vi "1C Camera Interpreter.vi"() -> (0 "error out":errorcluster, 1 "Overhead Image":T1(plugin-control), 2 "Heading":T2 format="%05.1f", 3 "Boat Location":T3, 4 "Time Elapsed (s)\nSince Last Image":dbl)   [LabVIEW 2011]
doc: "Using data from a cameram, attempts to track two fiducial patterns on the boat, one on the bow and one on the stern. Uses these positions to estimate boat position in the pool.\n\noptimizations for speed: \n-uses an oval-shaped mask to search for the tracking patterns only inside the pool\n-runs the two pattern searches separately so that they can be parallelized\n-upgraded to larger patterns\n\nBy: Cory Dolphin, Jason Curtis, Gray Thomas"
uses:
  <vilib>/userdefined/High Color/IMAQdx.ctl
  2-RIO/2 Typedefs/UTM Location.ctl
  2-RIO/2 Typedefs/heading.ctl
  2-RIO/2 Typedefs/indicator LED.ctl
  2-RIO/2 Globals/2 Global.vi
  <vilib>/vision/driver/NI_Vision_Acquisition_Software.lvlib
panel:
  out "Masked image":T1(plugin-control)
  in  "Minimum Stern Match Score":sgl=650.0
  in  "Minimum Bow Match Score":sgl=850.0
  in  "Reset Camera":bool
  in  "Camera Selector":T4="cam7"
  # "(ignore UTM Zone \nand Hemisphere for \nRC boat)"
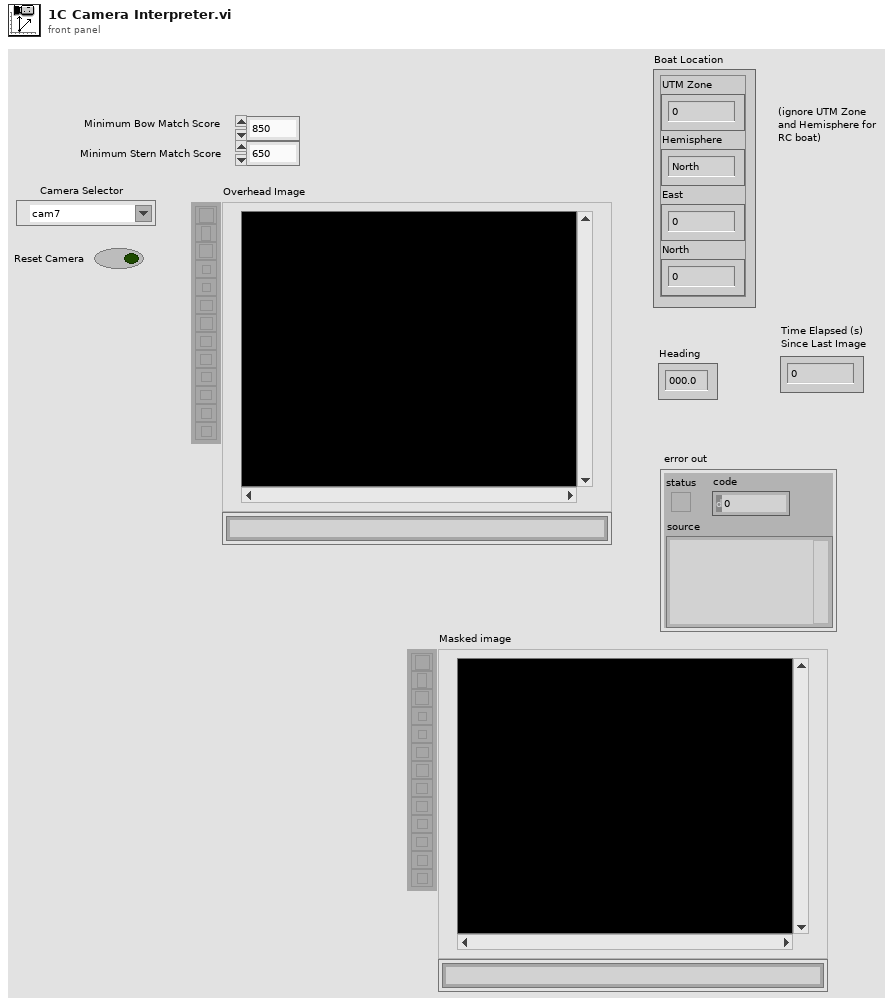
[diagram p1: front panel]
types:
  T1 = typedef "IMAQ Image.ctl" = refnum<image>
  T2 = typedef "heading.ctl" = dbl
  T3 = typedef "UTM Location.ctl" = cluster{"UTM Zone":dbl, "Hemisphere":enum16{"North", "South"}, "East":dbl, "North":dbl}
  T4 = typedef "IMAQdx.ctl" = refnum<k21>
  T5 = typedef "Image Type" = u32
  T6 = typedef "indicator LED.ctl" = bool
  T7 = typedef "generalized sensor status.ctl" = cluster{"Sensor Connected":T6, "Sensor Initialized":T6, "Sensor OK":T6, "Latest Error String":string}
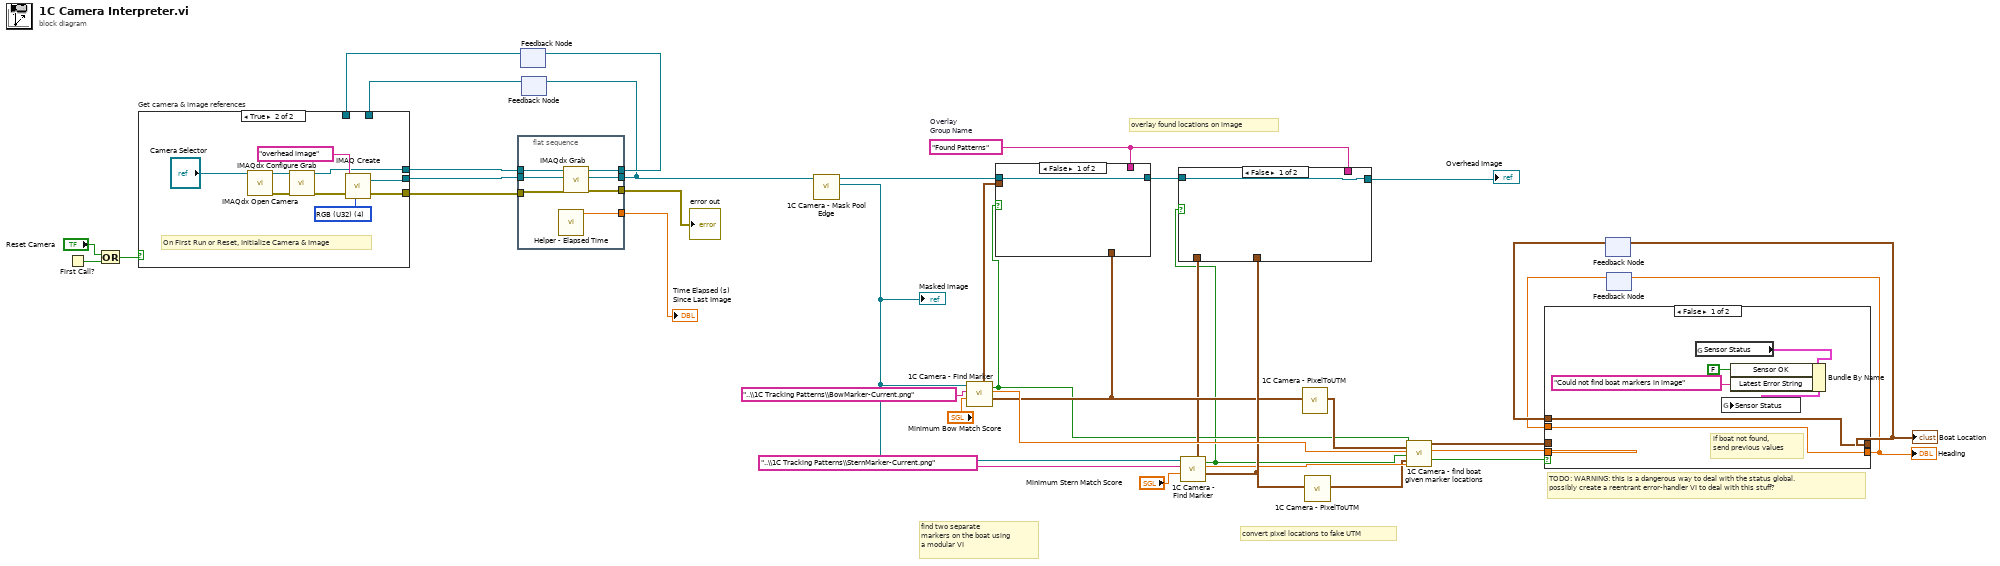
[diagram p0: block diagram]
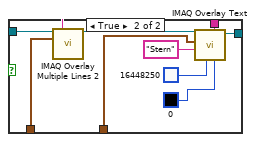
[diagram p2: hidden frame]
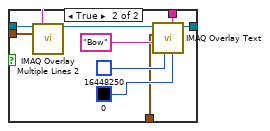
[diagram p3: hidden frame]
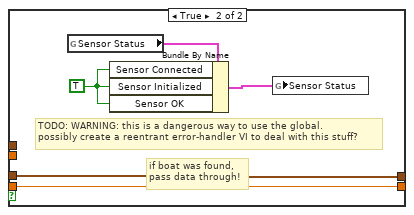
[diagram p4: hidden frame]
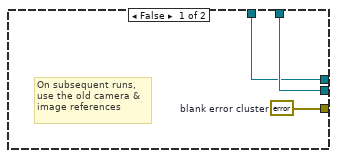
[diagram p5: hidden frame]
diagram:
  w7 = "Found Patterns"  # Overlay Group Name
  # "find two separate\nmarkers on the boat using \na modular VI"
  # "TODO: WARNING: this is a dangerous way to deal with the status global. \npossibly create a reentrant error-handler VI to deal with this stuff?"
  # "convert pixel locations to fake UTM"
  # "overlay found locations on image"
  n1 = First Call?() -> (First Call?: T/F=w37:bool)
  n2 = Or(x="Reset Camera", y=w37) -> (x .or. y?=w30:bool)
  n3 = flat-sequence {
    tunnel: [w45] -> w38
    tunnel: w36 -> [w44]
    tunnel: w35 -> [w43]
    tunnel: w34 -> [w42]
    tunnel: [w41] -> w33
    tunnel: [w40] -> w17
    tunnel: [w39] -> w6
    frame #0 {
      n4 = call "Helper - Elapsed Time.vi"() -> ("Time Elapsed (s)\nSince Last Iteration"=w39:dbl)  [unwired: 10 in, 1 out]
      n5 = call <vilib>:"IMAQdx Grab.vi"("error in"=w43, "Image In"=w42, "Session In"=w44) -> ("error out"=w45:errorcluster, "Image Out"=w40:T1, "Session Out"=w41:T4)  [unwired: 5 in, 1 out]
    }
  }
  n6 = feedback #1() -> (w31:T4)  [unwired: 1 in]
  n7 = feedback-in #1(w33) -> ()
  n8 = feedback-in #2(w17) -> ()
  n9 = feedback #2() -> (w32:T1)  [unwired: 1 in]
  n10 = case "Get camera & image references" shown="True" w30 {
    tunnel: [w47 w51] -> w36
    tunnel: [w46 w50] -> w35
    tunnel: [w48 w49] -> w34
    tunnel: w32 -> [w48 _]
    tunnel: w31 -> [w47 _]
    frame False {
      w46 = errorcluster {"status"=FALSE, "code"=0, "source"=""}  # blank error cluster
      # "On subsequent runs,\nuse the old camera &\nimage references"
    }
    frame True {
      w53 = T5 4 items=["Grayscale (U8)", "Grayscale (I16)", "Grayscale (SGL)", "Complex (CSG)", "RGB (U32)", "HSL (U32)", "RGB (U64)", "Grayscale (U16)"] ("Image Type")
      # "On First Run or Reset, Initialize Camera & Image"
      n11 = call <vilib>:"IMAQdx Open Camera.vi"("Session In"="Camera Selector") -> ("error out"=w54:errorcluster, "Session Out"=w57:T4)  [unwired: 9 in]
      n12 = call <vilib>:"IMAQdx Configure Grab.vi"("error in"=w54, "Session In"=w57) -> ("error out"=w55:errorcluster, "Session Out"=w51:T4)  [unwired: 8 in]
      n13 = call "IMAQ Create"("Image Name"="overhead image", "Image Type"=w53, "error in (no error)"=w55) -> ("New Image"=w49:T1, "error out"=w50:errorcluster)  [unwired: 2 in]
    }
  }
  n14 = call "1C Camera - Mask Pool Edge.vi"("Source Image In"=w17) -> ("Masked Image Out"=w1:T1, "Src Image Out"=w16:T1)  [unwired: 9 in]
  "Masked image" <- w1
  n15 = call "1C Camera - Find Marker.vi"("Minimum Match Score (650)"="Minimum Bow Match Score", "marker template relative path"="..\\1C Tracking Patterns\\BowMarker-Current.png", "Image In"=w1) -> ("Best Match Position"=w15:cluster{"x":sgl, "y":sgl}, "Best Match Heading"=w28:T2, "Best Match\nBounding Box"=w11:cluster{"x":sgl, "y":sgl}[], "Marker found?"=w5:T6)  [unwired: 3 in, 2 out]
  n16 = case shown="False" w5 {
    tunnel: w16 -> [w58 w64]
    tunnel: w15 -> [_ w63]
    tunnel: w11 -> [_ w61]
    tunnel: [w58 w60] -> w10
    tunnel: w7 -> [_ w59]
    frame False {
    }
    frame True {
      n17 = call "IMAQ Overlay Multiple Lines 2"("Image"=w64, "Group"=w59, "Line End Points"=w61) -> ("Image Out"=w62:T1)  [unwired: 11 in, 1 out]
      n18 = call "IMAQ Overlay Text"("BG Color (Transparent)"=u32 0, "Group"=w59, "Text Color (black)"=u32 16448250, "String"="Bow", "Origin"=w63, "Image"=w62) -> ("Image Out"=w60:T1)  [unwired: 4 in, 1 out]
    }
  }
  n19 = call "1C Camera - Find Marker.vi"("Minimum Match Score (650)"="Minimum Stern Match Score", "marker template relative path"="..\\1C Tracking Patterns\\SternMarker-Current.png", "Image In"=w1) -> ("Best Match Position"=w27:cluster{"x":sgl, "y":sgl}, "Best Match Heading"=w14:T2, "Best Match\nBounding Box"=w9:cluster{"x":sgl, "y":sgl}[], "Marker found?"=w4:T6)  [unwired: 3 in, 2 out]
  n20 = case shown="False" w4 {
    tunnel: w27 -> [_ w74]
    tunnel: w10 -> [w68 w73]
    tunnel: w9 -> [_ w71]
    tunnel: [w68 w70] -> w8
    tunnel: w7 -> [_ w69]
    frame False {
    }
    frame True {
      n21 = call "IMAQ Overlay Multiple Lines 2"("Image"=w73, "Group"=w69, "Line End Points"=w71) -> ("Image Out"=w72:T1)  [unwired: 11 in, 1 out]
      n22 = call "IMAQ Overlay Text"("BG Color (Transparent)"=u32 0, "Group"=w69, "Text Color (black)"=u32 16448250, "String"="Stern", "Origin"=w74, "Image"=w72) -> ("Image Out"=w70:T1)  [unwired: 4 in, 1 out]
    }
  }
  "Overhead Image" <- w8
  n23 = call "1C Camera - PixelToUTM.vi"("Found Marker Position in (pixels)"=w15) -> ("UTM Location Out"=w13:T3)  [unwired: 10 in]
  n24 = call "1C Camera - PixelToUTM.vi"("Found Marker Position in (pixels)"=w27) -> ("UTM Location Out"=w12:T3)  [unwired: 10 in]
  n25 = call "1C Camera - find boat given marker locations.vi"("Bow Marker Found"=w5, "Bow Marker Location"=w13, "Bow Marker Heading"=w28, "Stern Marker Found"=w4, "Stern Marker Location"=w12, "Stern Marker Heading"=w14) -> ("Boat Location"=w25:T3, "Heading"=w24:T2, "Boat Found"=w26:T6)  [unwired: 11 in]
  n26 = feedback #3() -> (w22:T3)  [unwired: 1 in]
  n27 = feedback #4() -> (w20:T2)  [unwired: 1 in]
  n28 = case shown="False" w26 {
    tunnel: [w83 w88] -> w23
    tunnel: w25 -> [_ w88]
    tunnel: [w82 w87] -> w21
    tunnel: w24 -> [_ w87]
    tunnel: w22 -> [w83 _]
    tunnel: w20 -> [w82 _]
    frame False {
      # "if boat not found,\nsend previous values"
      n29 = global read "2 Global.vi" "Sensor Status"() -> (w81:T7)
      n30 = Bundle By Name(cluster=w81, "Sensor OK"=T6 FALSE, "Latest Error String"="Could not find boat markers in image" ("Error String")) -> (w78:T7)
      n31 = global write "2 Global.vi" "Sensor Status"(w78) -> ()
    }
    frame True {
      w84 = T6 TRUE ("Sensor OK")
      # "TODO: WARNING: this is a dangerous way to use the global. \npossibly create a reentrant error-handler VI to deal with this stuff?"
      # "if boat was found, \npass data through!"
      n32 = global read "2 Global.vi" "Sensor Status"() -> (w86:T7)
      n33 = Bundle By Name(cluster=w86, "Sensor Connected"=w84, "Sensor Initialized"=w84, "Sensor OK"=w84) -> (w85:T7)
      n34 = global write "2 Global.vi" "Sensor Status"(w85) -> ()
    }
  }
  "Boat Location" <- w23
  "Heading" <- w21
  n35 = feedback-in #3(w23) -> ()
  n36 = feedback-in #4(w21) -> ()
  "error out" <- w38
  "Time Elapsed (s)\nSince Last Image" <- w6
